vi "836_MultiCameraIPCameraRead.vi"(0 "Refnum in":T1, 1 "Operation":enum16{"Read", "Reopen", "Close"}(ring), 5 "address":string, 7 "Camera Settings":T2, 9 "millisecond timer value in":u32, 11 "error in (no error)":errorcluster, 12 "Numeric in":i32) -> (4 "Refnum out":T1, 6 "Numeric 3":i32, 8 "Numeric out":i32, 10 "millisecond timer value out":u32, 15 "error out":errorcluster)   [LabVIEW 2015]
uses:
  <vilib>/Rock Robotics/WPI/Camera/WPI_CameraSettings Read MJPG.ctl
  <vilib>/Rock Robotics/WPI/Camera/WPI_CameraImageSize.ctl
  <vilib>/vision/Image Controls.llb/IMAQ Image.ctl
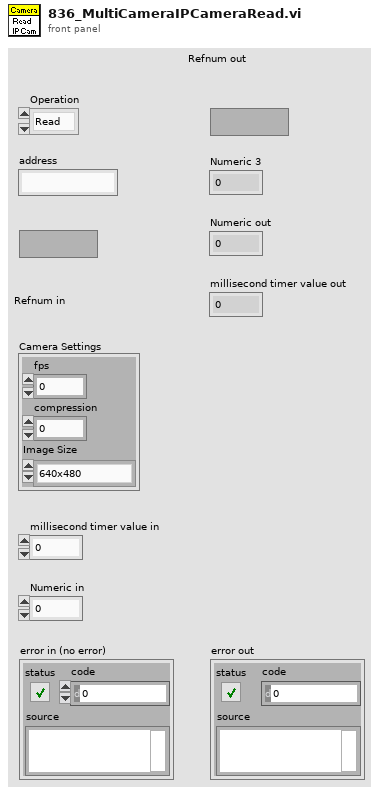
[diagram p1: front panel]
types:
  T1 = typedef "IMAQ Image.ctl" = refnum<image>
  T2 = typedef "WPI_CameraSettings Read MJPG.ctl" = cluster{"fps":i32, "compression":i32, "Image Size":T3}
  T3 = typedef "WPI_CameraImageSize.ctl" = enum16{"640x480", "320x240", "160x120", "Custom"}
  T4 = enum16{"Standard", "Buffered", "CRLF", "Immediate"}
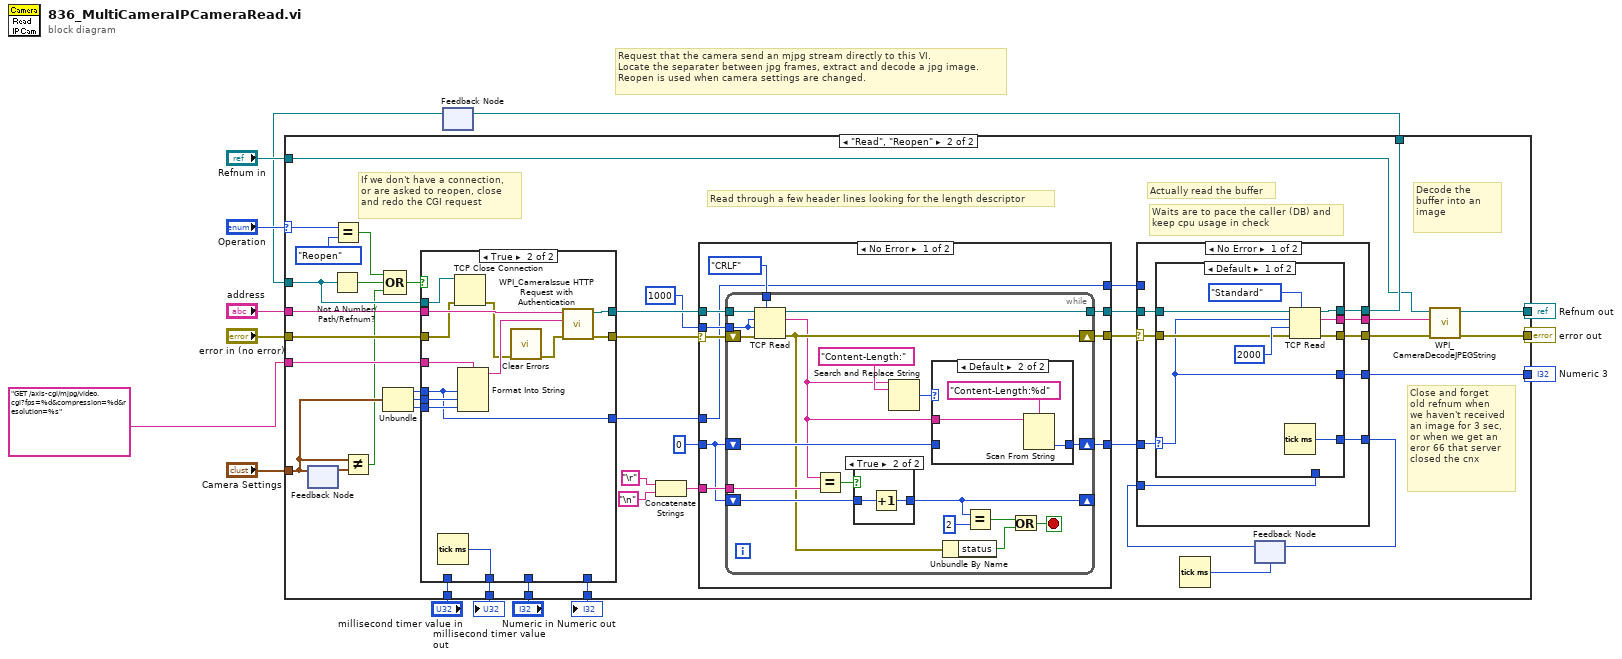
[diagram p0: block diagram]
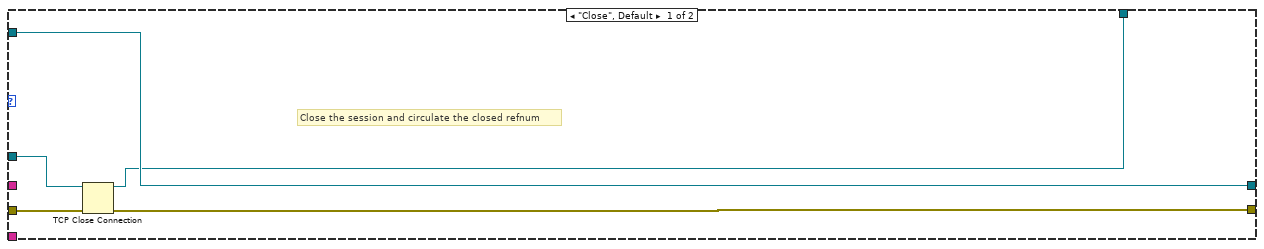
[diagram p2: hidden frame]
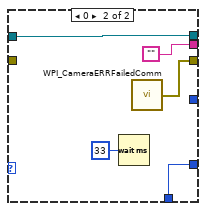
[diagram p4: hidden frame]
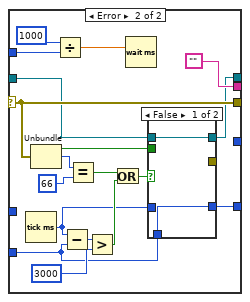
[diagram p5: hidden frame]
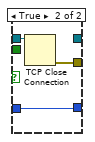
[diagram p6: hidden frame]
diagram:
  # "Request that the camera send an mjpg stream directly to this VI.\nLocate the separater between jpg frames, extract and decode a jpg image.\nReopen is used when camera settings are changed."
  n1 = feedback #1() -> (w7:refnum<k5>)  [unwired: 1 out]
  n2 = case shown="\"Read\", \"Reopen\"" "Operation" {
    selector: "Operation" -> [_ w39]
    tunnel: "error in (no error)" -> [w19 w52]
    tunnel: "address" -> [_ w51]
    tunnel: [w16 w50] -> w4
    tunnel: "GET /axis-cgi/mjpg/video.cgi?fps=%d&compression=%d&resolution=%s" -> [_ w49]
    tunnel: "Camera Settings" -> [_ w27]
    tunnel: [w17 w44] -> w5
    tunnel: [w18 w42] -> w6
    tunnel: w7 -> [w20 w40]
    tunnel: "Refnum in" -> [w17 w38]
    tunnel: [_ w33] -> w10
    tunnel: "Numeric in" -> [_ w32]
    tunnel: [_ w31] -> w12
    tunnel: "millisecond timer value in" -> [_ w30]
    tunnel: [_ w29] -> w14
    frame "Close", Default {
      # "Close the session and circulate the closed refnum"
      n3 = TCP Close Connection(connection ID=w20, error in (no error)=w19) -> (connection ID out=w16:refnum<k5>, error out=w18:errorcluster)  [unwired: 1 out]
    }
    frame "Read", "Reopen" {
      # "Waits are to pace the caller (DB) and\nkeep cpu usage in check"
      # "Close and forget\nold refnum when\nwe haven't received\nan image for 3 sec,\nor when we get an\neror 66 that server\nclosed the cnx"
      # "Decode the buffer into an image"
      # "Actually read the buffer"
      # "Read through a few header lines looking for the length descriptor"
      # "If we don't have a connection,\nor are asked to reopen, close\nand redo the CGI request"
      n4 = feedback #2() -> (w28:T2)  [unwired: 1 out]
      n5 = feedback-in #2(w27) -> ()
      n6 = Not A Number/Path/Refnum?(number/path/refnum=w40) -> (NaN/Path/Refnum?=w25:bool)
      n7 = Equal?(x=w39, y=enum16{"Read", "Reopen", "Close"}."Reopen" ("Operation")) -> (x = y?=w26:bool)
      n8 = Not Equal?(x=w27, y=w28) -> (x != y?=w23:bool)
      n9 = Unbundle(w27) -> ("fps"=w46:i32, "compression"=w45:i32, "Image Size"=w37:T3)
      n10 = Compound Arithmetic op=OR(w26, w25, w23) -> (w24:bool)
      n11 = case shown="True" w24 {
        tunnel: [w65 w74] -> w56
        tunnel: [w66 w75] -> w55
        tunnel: w52 -> [w65 w72]
        tunnel: w51 -> [_ w77]
        tunnel: w40 -> [w66 w73]
        tunnel: w49 -> [_ w79]
        tunnel: w46 -> [w62 w67]
        tunnel: w45 -> [_ w78]
        tunnel: w37 -> [_ w69]
        tunnel: w32 -> [w64 _]
        tunnel: [w64 _] -> w31
        tunnel: w30 -> [w63 _]
        tunnel: [w63 w68] -> w29
        tunnel: [w62 w67] -> w21
        frame False {
        }
        frame True {
          n12 = Tick Count (ms)() -> (millisecond timer value=w68:u32)
          n13 = TCP Close Connection(connection ID=w73, error in (no error)=w72) -> (error out=w71:errorcluster)  [unwired: 2 out]
          n14 = Format Into String(format string=w79, w67, w78, w69) -> (resulting string=w76:string)  [unwired: 2 in, 1 out]
          n15 = call <vilib>:"Clear Errors.vi"("error in (no error)"=w71) -> ("error out"=w70:errorcluster)  [unwired: 1 in, 5 out]
          n16 = call <vilib>:"WPI_CameraIssue HTTP Request with Authentication.vi"("error in (no error)"=w70, "Request"=w76, "address"=w77) -> ("error out"=w74:errorcluster, "connection ID (dup)"=w75:refnum<k5>)  [unwired: 7 out]
        }
      }
      n17 = Concatenate Strings("\r", "\n") -> (w59:string)
      n18 = case shown="No Error" w56 {
        selector: w56 -> [w128 w164]
        tunnel: [w135 w164] -> w53
        tunnel: [w134 w163] -> w58
        tunnel: [w133 w165] -> w57
        tunnel: w59 -> [w132 _]
        tunnel: w55 -> [w130 w165]
        tunnel: 1000 ("bytes to read") -> [w129 _]
        tunnel: 0 -> [w127 w163]
        tunnel: [w126 w162] -> w22
        tunnel: w21 -> [w126 w162]
        frame No Error {
          n19 = while {
            tunnel: w130 -> [w154]
            tunnel: [w153] -> w133
            shift-right: [w152] -> w134
            shift-left: w127 -> [w151]
            shift-right: [w148] -> _
            shift-left: w127 -> [w149]
            tunnel: w132 -> [w146]
            tunnel: w129 -> [w136]
            tunnel: T4."CRLF" ("mode (standard)") -> [w145]
            shift-right: [w143] -> w135
            shift-left: w128 -> [w144]
            stop <- w142 stop-if-true
            n20 = TCP Read(connection ID=w154, bytes to read=w136, error in (no error)=w144, 7:w145, 9:w136) -> (connection ID out=w153:refnum<k5>, data out=w137:string, error out=w143:errorcluster)
            n21 = Equal?(x=w137, y=w146) -> (x = y?=w150:bool)
            n22 = case shown="True" w150 {
              tunnel: w149 -> [w155 w157]
              tunnel: [w155 w156] -> w148
              frame False {
              }
              frame True {
                n23 = Increment(x=w157) -> (x+1=w156:i32)
              }
            }
            n24 = Search and Replace String(input string=w137, search string="Content-Length:" ("regular expression")) -> (number of replacements=w141:i32)  [unwired: 1 in, 8 out]
            n25 = case shown="Default" w141 {
              tunnel: [w158 w161] -> w152
              tunnel: w151 -> [w158 _]
              tunnel: w137 -> [_ w160]
              frame 0 {
              }
              frame Default {
                n26 = Scan From String(format string="Content-Length:%d" ("regular expression"), input string=w160) -> (output 1=w161:i32)  [unwired: 2 in, 4 out]
              }
            }
            n27 = Unbundle By Name(w143) -> ("status"=w138:bool)
            n28 = Equal?(x=w148, y=2) -> (x = y?=w139:bool)
            n29 = Or(x=w139, y=w138) -> (x .or. y?=w142:bool)
          }
        }
        frame Error {
        }
      }
      n30 = Tick Count (ms)() -> (millisecond timer value=w35:u32)
      n31 = feedback #3(w35) -> (w34:u32)
      n32 = case shown="No Error" w53 {
        selector: w53 -> [w84 w119]
        tunnel: [w88 w119] -> w43
        tunnel: [w87 ""] -> w47
        tunnel: [w86 w116] -> w50
        tunnel: w58 -> [w83 _]
        tunnel: w57 -> [w85 w117]
        tunnel: [w82 w108] -> w36
        tunnel: w34 -> [w81 w106]
        tunnel: [w80 _] -> w33
        tunnel: w22 -> [_ w103]
        frame No Error {
          n33 = case shown="Default" w83 {
            selector: w83 -> [w89 _]
            tunnel: w85 -> [w97 w101]
            tunnel: [w96 w100] -> w88
            tunnel: [w93 ""] -> w87
            tunnel: [w92 w101] -> w86
            tunnel: w84 -> [w91 _]
            tunnel: [w90 w98] -> w82
            tunnel: w81 -> [_ w98]
            tunnel: [w89 _] -> w80
            frame Default {
              n34 = Tick Count (ms)() -> (millisecond timer value=w90:u32)
              n35 = TCP Read(connection ID=w97, bytes to read=w89, error in (no error)=w91, 7:T4."Standard" ("mode (standard)"), 9:2000 ("timeout ms (25000)")) -> (connection ID out=w92:refnum<k5>, data out=w93:string, error out=w96:errorcluster)
            }
            frame 0 {
              n36 = Wait (ms)(milliseconds to wait=u32 33) -> ()  [unwired: 1 out]
              n37 = call <vilib>:"WPI_CameraERRFailedComm.vi"() -> ("error out"=w100:errorcluster)
            }
          }
        }
        frame Error {
          n38 = Tick Count (ms)() -> (millisecond timer value=w107:u32)
          n39 = Unbundle(w119) -> ("status"=w118:bool, "code"=w114:i32)  [unwired: 1 out]
          n40 = Divide(x=u32 1000 ("milliseconds to wait"), y=w103) -> (x/y=w104:dbl)
          n41 = Subtract(x=w107, y=w106) -> (x-y=w109:u32)
          n42 = Equal?(x=w114, y=u32 66 ("milliseconds to wait")) -> (x = y?=w113:bool)
          n43 = Greater?(x=w109, y=u32 3000 ("milliseconds to wait")) -> (0:w111:bool)
          n44 = Or(x=w113, y=w111) -> (x .or. y?=w112:bool)
          n45 = Wait (ms)(milliseconds to wait=w104) -> ()  [unwired: 1 out]
          n46 = case shown="False" w112 {
            tunnel: w118 -> [_ _]
            tunnel: w117 -> [w122 w125]
            tunnel: [w122 _] -> w116
            tunnel: [w121 w124] -> w108
            tunnel: w107 -> [_ w124]
            tunnel: w106 -> [w121 _]
            tunnel: [_ w123] -> _
            frame False {
            }
            frame True {
              n47 = TCP Close Connection(connection ID=w125) -> (error out=w123:errorcluster)  [unwired: 1 in, 2 out]
            }
          }
        }
      }
      n48 = feedback-in #3(w36) -> ()
      n49 = call <vilib>:"WPI_CameraDecodeJPEGString.vi"("error in"=w43, "Compressed Image"=w47, "Image In"=w38) -> ("error out"=w42:errorcluster, "Image Out"=w44:T1)  [unwired: 3 out]
    }
  }
  "millisecond timer value out" <- w14
  "Numeric out" <- w12
  "Numeric 3" <- w10
  "error out" <- w6
  "Refnum out" <- w5
  n50 = feedback-in #1(w4) -> ()
